vi "Read_Numato_Relays.vi"(8 "error in (no error)":errorcluster) -> (0 "error out":errorcluster, 3 "Relays":T1)   [LabVIEW 2025]
uses:
  Controls/DUT_Relays.ctl
  Controls/CHMB_Relays.ctl
  Controls/Relays.ctl
  <vilib>/Utility/config.llb/Read Key (U32).vi
  <vilib>/Utility/config.llb/NI_LVConfig.lvlib
panel:
  out "CHMB2":T2
  out "CHMB1":T2
  out "DUT4":T3
  out "DUT3":T3
  out "DUT2":T3
  out "DUT1":T3
  out "error IO":errorcluster
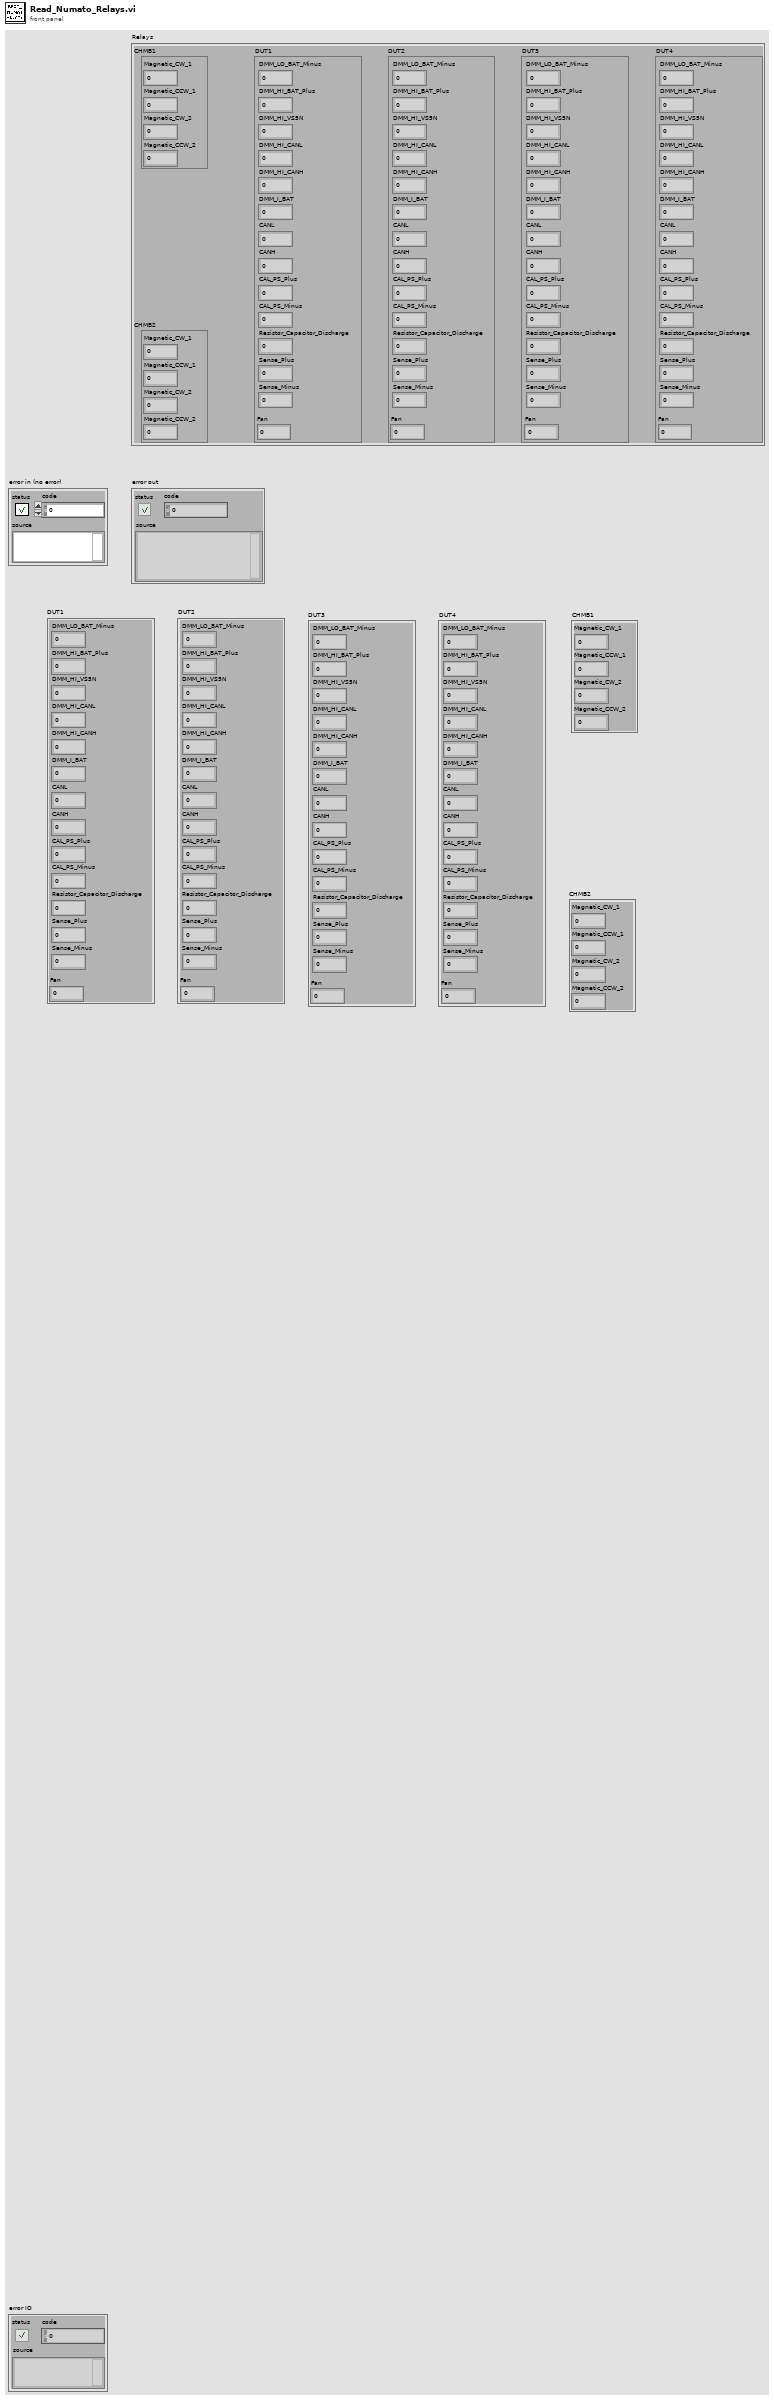
[diagram p1: front panel]
types:
  T1 = typedef "Relays.ctl" = cluster{"CHMB1":T2, "CHMB2":T2, "DUT1":T3, "DUT2":T3, "DUT3":T3, "DUT4":T3}
  T2 = typedef "CHMB_Relays.ctl" = cluster{"Magnetic_CW_1":i32, "Magnetic_CCW_1":i32, "Magnetic_CW_2":i32, "Magnetic_CCW_2":i32}
  T3 = typedef "DUT_Relays.ctl" = cluster{"DMM_LO_BAT_Minus":i32, "DMM_HI_BAT_Plus":i32, "DMM_HI_VS5N":i32, "DMM_HI_CANL":i32, "DMM_HI_CANH":i32, "DMM_I_BAT":i32, "CANL":i32, "CANH":i32, "CAL_PS_Plus":i32, "CAL_PS_Minus":i32, "Resistor_Capacitor_Discharge":i32, "Sense_Plus":i32, "Sense_Minus":i32, "Fan":i32}
  T4 = typedef "NI_LVConfig.lvlib/Config Data RefNum.ctl" = refnum<k1>
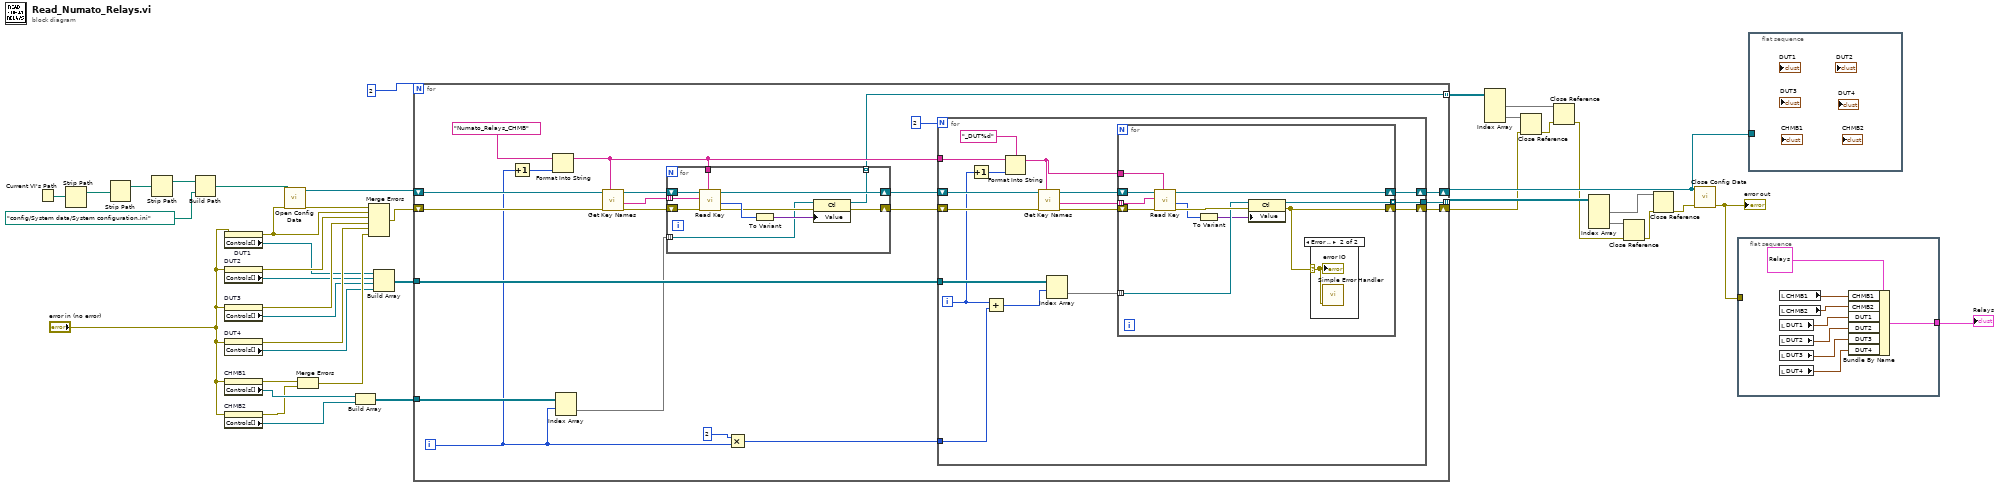
[diagram p0: block diagram]
diagram:
  n1 = Current VI's Path() -> (path=w28:path)
  n2 = Strip Path(path=w28) -> (stripped path=w27:path)  [unwired: 1 out]
  n3 = Strip Path(path=w27) -> (stripped path=w31:path)  [unwired: 1 out]
  n4 = Strip Path(path=w31) -> (stripped path=w30:path)  [unwired: 1 out]
  n5 = Build Path(base path=w30, name or relative path=path "config/System data/System configuration.ini") -> (appended path=w26:path)
  n6 = property on="DUT1" class="Clust (strict)"(error in="error in (no error)") -> (error out=w25:errorcluster, "Controls[]"=w19:refnum<vi>[])  [unwired: 1 in, 1 out]
  n7 = property on="DUT2" class="Clust (strict)"(error in="error in (no error)") -> (error out=w24:errorcluster, "Controls[]"=w18:refnum<vi>[])  [unwired: 1 in, 1 out]
  n8 = property on="DUT3" class="Clust (strict)"(error in="error in (no error)") -> (error out=w22:errorcluster, "Controls[]"=w17:refnum<vi>[])  [unwired: 1 in, 1 out]
  n9 = property on="DUT4" class="Clust (strict)"(error in="error in (no error)") -> (error out=w21:errorcluster, "Controls[]"=w16:refnum<vi>[])  [unwired: 1 in, 1 out]
  n10 = property on="CHMB1" class="Clust (strict)"(error in="error in (no error)") -> (error out=w23:errorcluster, "Controls[]"=w14:refnum<vi>[])  [unwired: 1 in, 1 out]
  n11 = property on="CHMB2" class="Clust (strict)"(error in="error in (no error)") -> (error out=w7:errorcluster, "Controls[]"=w6:refnum<vi>[])  [unwired: 1 in, 1 out]
  n12 = call <vilib>:"Open Config Data.vi"("error in (no error)"=w25, "configuration file path"=w26) -> ("error out"=w36:errorcluster, "refnum"=w40:T4)  [unwired: 7 in, 1 out]
  n13 = Merge Errors(w23, w7) -> (w20:errorcluster)
  n14 = Build Array(w14, w6) -> (w13:refnum<vi>[][])
  n15 = Merge Errors(w36, w25, w24, w22, w21, w20) -> (w38:errorcluster)
  n16 = Build Array(w19, w18, w17, w16) -> (w15:refnum<vi>[][])
  n17 = for {
    N: 2 -> [_]
    shift-right: [w60] -> w5
    shift-left: w40 -> [w56]
    shift-right: [w61] -> w4
    shift-left: w38 -> [w55]
    tunnel: [w58] -> w35 mode=indexing
    tunnel: w15 -> [w53]
    tunnel: w13 -> [w51]
    tunnel: [w42] -> w12 mode=indexing
    i -> [w41]
    n18 = Increment(x=w41) -> (x+1=w52:i32)
    n19 = Format Into String(initial string="Numato_Relays_CHMB" ("section"), w52) -> (resulting string=w47:string)  [unwired: 2 in, 1 out]
    n20 = Index Array(array=w51, index (row)=w41) -> (element=w50:refnum<vi>[])  [unwired: 1 in]
    n21 = call <vilib>:"Get Key Names.vi"("section"=w47, "error in (no error)"=w55, "refnum"=w56) -> ("error out"=w45:errorcluster, "key names"=w54:string[], "refnum out"=w44:T4)  [unwired: 5 in, 1 out]
    n22 = for {
      tunnel: w54 -> [w69] mode=indexing
      tunnel: w50 -> [w67] mode=indexing
      tunnel: w47 -> [w68]
      shift-right: [w66] -> w46
      shift-left: w45 -> [w62]
      shift-right: [w64] -> w43
      shift-left: w44 -> [w65]
      tunnel: [w63] -> w42 mode=indexing
      n23 = call-poly <vilib>:"Read Key.vi"("section"=w68, "error in (no error)"=w62, "key"=w69, "refnum"=w65) -> ("error out"=w70:errorcluster, "value"=w71:u32, "refnum out"=w64:T4)  [unwired: 4 in, 1 out]
      n24 = To Variant(anything=w71) -> (Variant=w72:variant)
      n25 = property class="Ctl"(reference=w67, error in=w70, "Value"=w72) -> (reference out=w63:refnum<vi>, error out=w66:errorcluster)
    }
    n26 = Multiply(x=2, y=w41) -> (x*y=w48:i32)
    n27 = for {
      N: 2 -> [_]
      tunnel: [w83] -> w58
      shift-right: [w84] -> w60
      shift-left: w43 -> [w89]
      shift-right: [w85] -> w61
      shift-left: w46 -> [w87]
      tunnel: w47 -> [w81]
      tunnel: w53 -> [w78]
      tunnel: w48 -> [w75]
      i -> [w73]
      n28 = Increment(x=w73) -> (x+1=w76:i32)
      n29 = Add(x=w73, y=w75) -> (x+y=w74:i32)
      n30 = Format Into String(format string="_DUT%d", initial string=w81, w76) -> (resulting string=w80:string)  [unwired: 1 in, 1 out]
      n31 = call <vilib>:"Get Key Names.vi"("section"=w80, "error in (no error)"=w87, "refnum"=w89) -> ("error out"=w86:errorcluster, "key names"=w82:string[], "refnum out"=w88:T4)  [unwired: 5 in, 1 out]
      n32 = Index Array(array=w78, index (row)=w74) -> (element=w77:refnum<vi>[])  [unwired: 1 in]
      n33 = for {
        tunnel: w82 -> [w98] mode=indexing
        shift-right: [w99] -> w84
        shift-left: w88 -> [w100]
        tunnel: w80 -> [w97]
        tunnel: [w94] -> w83 mode=indexing
        shift-right: [w93] -> w85
        shift-left: w86 -> [w96]
        tunnel: w77 -> [w91] mode=indexing
        n34 = call-poly <vilib>:"Read Key.vi"("section"=w97, "error in (no error)"=w96, "key"=w98, "refnum"=w100) -> ("error out"=w95:errorcluster, "value"=w92:u32, "refnum out"=w99:T4)  [unwired: 4 in, 1 out]
        n35 = To Variant(anything=w92) -> (Variant=w90:variant)
        n36 = property class="Ctl"(reference=w91, error in=w95, "Value"=w90) -> (reference out=w94:refnum<vi>, error out=w93:errorcluster)
        n37 = case shown="Error .." w93 {
          selector: w93 -> [_ w101]
          frame No Error {
          }
          frame Error {
            n38 = call <vilib>:"Simple Error Handler.vi"("error in (no error)"=w101) -> ()  [unwired: 4 in, 5 out]
            "error IO" <- w101
          }
        }
      }
    }
  }
  n39 = Index Array(array=w12) -> (element #1=w9:refnum<vi>[], element #2=w10:refnum<vi>[])  [unwired: 4 in]
  n40 = Close Reference(reference=w10, error in (no error)=w4) -> (error out=w11:errorcluster)
  n41 = Close Reference(reference=w9, error in (no error)=w11) -> (error out=w2:errorcluster)
  n42 = Index Array(array=w35) -> (element #1=w34:refnum<vi>[], element #2=w33:refnum<vi>[])  [unwired: 4 in]
  n43 = Close Reference(reference=w33, error in (no error)=w2) -> (error out=w32:errorcluster)
  n44 = Close Reference(reference=w34, error in (no error)=w32) -> (error out=w39:errorcluster)
  n45 = call <vilib>:"Close Config Data.vi"("error in (no error)"=w39, "refnum"=w5) -> ("error out"=w1:errorcluster)  [unwired: 8 in, 1 out]
  "error out" <- w1
  n46 = flat-sequence {
    tunnel: w1 -> [_]
    tunnel: [w103] -> w3
    frame #0 {
      n47 = local read "CHMB1"() -> (w108:T2)
      n48 = local read "CHMB2"() -> (w102:T2)
      n49 = local read "DUT1"() -> (w107:T3)
      n50 = local read "DUT2"() -> (w106:T3)
      n51 = local read "DUT3"() -> (w105:T3)
      n52 = local read "DUT4"() -> (w104:T3)
      n53 = Bundle By Name(cluster=T1 {"CHMB1"={"Magnetic_CW_1"=0, "Magnetic_CCW_1"=0, "Magnetic_CW_2"=0, "Magnetic_CCW_2"=0}, "CHMB2"={"Magnetic_CW_1"=0, "Magnetic_CCW_1"=0, "Magnetic_CW_2"=0, "Magnetic_CCW_2"=0}, "DUT1"={"DMM_LO_BAT_Minus"=0, "DMM_HI_BAT_Plus"=0, "DMM_HI_VS5N"=0, "DMM_HI_CANL"=0, "DMM_HI_CANH"=0, "DMM_I_BAT"=0, "CANL"=0, "CANH"=0, "CAL_PS_Plus"=0, "CAL_PS_Minus"=0, "Resistor_Capacitor_Discharge"=0, "Sense_Plus"=0, "Sense_Minus"=0, "Fan"=0}, "DUT2"={"DMM_LO_BAT_Minus"=0, "DMM_HI_BAT_Plus"=0, "DMM_HI_VS5N"=0, "DMM_HI_CANL"=0, "DMM_HI_CANH"=0, "DMM_I_BAT"=0, "CANL"=0, "CANH"=0, "CAL_PS_Plus"=0, "CAL_PS_Minus"=0, "Resistor_Capacitor_Discharge"=0, "Sense_Plus"=0, "Sense_Minus"=0, "Fan"=0}, "DUT3"={"DMM_LO_BAT_Minus"=0, "DMM_HI_BAT_Plus"=0, "DMM_HI_VS5N"=0, "DMM_HI_CANL"=0, "DMM_HI_CANH"=0, "DMM_I_BAT"=0, "CANL"=0, "CANH"=0, "CAL_PS_Plus"=0, "CAL_PS_Minus"=0, "Resistor_Capacitor_Discharge"=0, "Sense_Plus"=0, "Sense_Minus"=0, "Fan"=0}, "DUT4"={"DMM_LO_BAT_Minus"=0, "DMM_HI_BAT_Plus"=0, "DMM_HI_VS5N"=0, "DMM_HI_CANL"=0, "DMM_HI_CANH"=0, "DMM_I_BAT"=0, "CANL"=0, "CANH"=0, "CAL_PS_Plus"=0, "CAL_PS_Minus"=0, "Resistor_Capacitor_Discharge"=0, "Sense_Plus"=0, "Sense_Minus"=0, "Fan"=0}} ("Relays"), "CHMB1"=w108, "CHMB2"=w102, "DUT1"=w107, "DUT2"=w106, "DUT3"=w105, "DUT4"=w104) -> (w103:T1)
    }
  }
  n54 = flat-sequence {
    tunnel: w5 -> [_]
    frame #0 {
    }
  }
  "Relays" <- w3
